vi "Calibration and Function folders.vi"(4 "ini file index":i64, 5 "Folder":T1) -> (2 "error out":errorcluster, 3 "Selected Folder":path)   [LabVIEW 2015]
uses:
  Calibration and Function folders.ctl
  <vilib>/Utility/sysdir.llb/System Directory Type.ctl
panel:
  out "All Files in Dir":path[](array[path])
  out "appended path":path
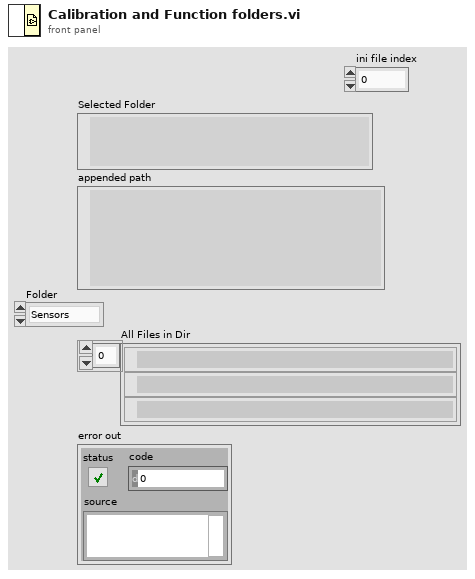
[diagram p1: front panel]
types:
  T1 = typedef "Calibration and Function folders.ctl" = enum16{"Sensors", "Functions", "Config File", "PublicAppFolder", "New ini File", "Set Config File", "Delete ini File"}
  T2 = enum16{"open", "replace", "create", "open or create", "replace or create", "replace or create with confirmation"}
  T3 = typedef "System Directory Type.ctl" = i32
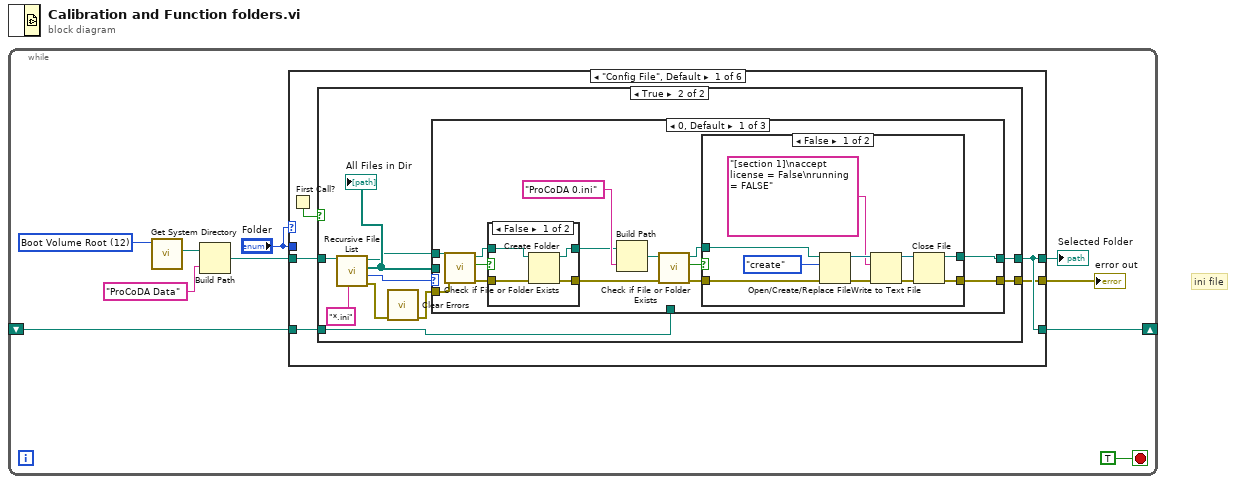
[diagram p0: block diagram]
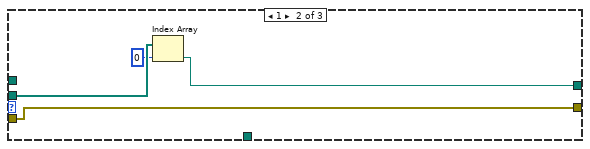
[diagram p5: hidden frame]
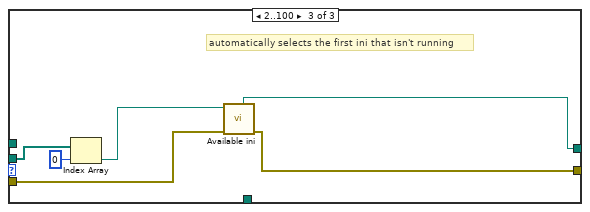
[diagram p6: hidden frame]
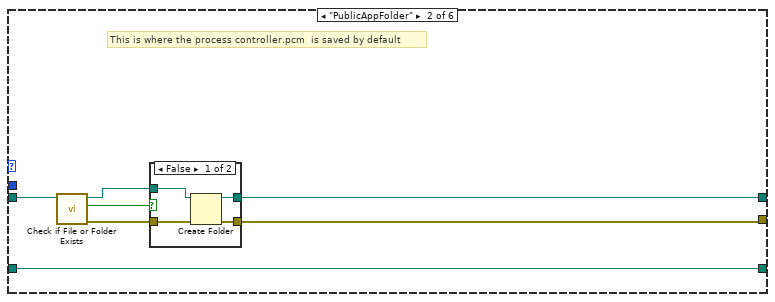
[diagram p7: hidden frame]
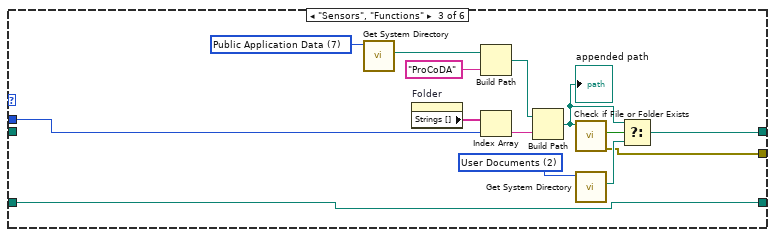
[diagram p9: hidden frame]
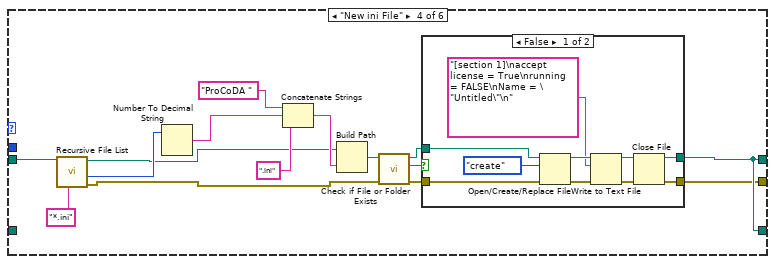
[diagram p10: hidden frame]
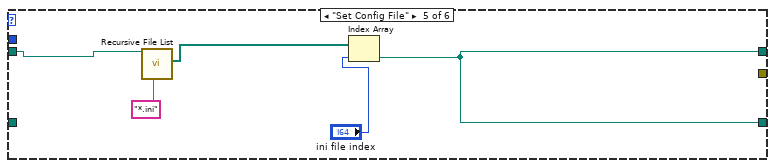
[diagram p12: hidden frame]
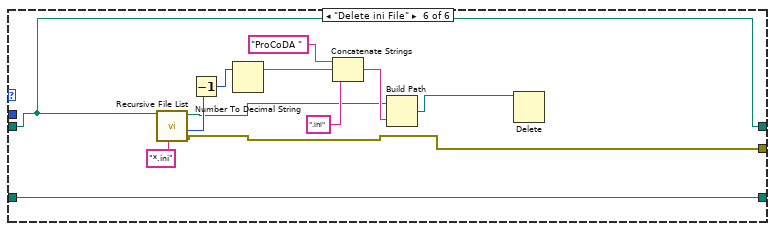
[diagram p13: hidden frame]
diagram:
  # "ini file"
  n1 = while {
    shift-right: [w3] -> _
    shift-left: _ -> [w2]
    stop <- TRUE stop-if-true
    w6 = T3 12 items=["User Home"=0, "User Desktop"=1, "User Documents"=2, "User Application Data"=3, "User Preferences"=4, "User Temporary"=5, "Public Documents"=6, "Public Application Data"=7, "Public Preferences"=8, "Public Cache"=13, "System Core Libraries"=9, "System Installed Libraries"=10, "Application Files"=11, "Boot Volume Root"=12] ("system directory type")
    n2 = call <vilib>:"Get System Directory.vi"("system directory type"=w6) -> ("system directory"=w8:path)  [unwired: 10 in]
    n3 = Build Path(base path=w8, name or relative path="ProCoDA Data") -> (appended path=w5:path)
    n4 = case shown="\"Config File\", Default" "Folder" {
      tunnel: [w14 w72 w90 w108 w123 w128] -> w10
      tunnel: "Folder" -> [_ _ w88 _ _ _]
      tunnel: w5 -> [w15 w71 _ w110 w126 w128]
      tunnel: [w14 w70 w83 w108 w123 w129] -> w3
      tunnel: w2 -> [w12 w70 w83 _ _ w129]
      tunnel: [w13 w69 w82 w107 _ w132] -> w1
      frame "Config File", Default {
        n5 = First Call?() -> (First Call?: T/F=w11:bool)
        n6 = case shown="True" w11 {
          tunnel: w15 -> [_ w26]
          tunnel: [w16 w23] -> w14
          tunnel: [_ w21] -> w13
          tunnel: w12 -> [w16 w18]
          frame False {
          }
          frame True {
            n7 = call <vilib>:"Recursive File List.vi"("pattern"="*.ini", "Folder Path"=w26) -> ("error out"=w19:errorcluster, "Number of Files"=w22:i32, "All Files in Dir"=w24:path[], "dup Folder Path"=w20:path)  [unwired: 5 in, 1 out]
            "All Files in Dir" <- w24
            n8 = call <vilib>:"Clear Errors.vi"("error in (no error)"=w19) -> ("error out"=w17:errorcluster)  [unwired: 5 in, 1 out]
            n9 = case shown="0, Default" w22 {
              tunnel: w24 -> [_ w62 w65]
              tunnel: [w30 w60 w68] -> w23
              tunnel: [w29 w59 w66] -> w21
              tunnel: w20 -> [w28 _ _]
              tunnel: w17 -> [w27 w59 w67]
              tunnel: w18 -> [_ _ _]
              frame 0, Default {
                n10 = call <vilib>:"Check if File or Folder Exists.vi"("error in (no error)"=w27, "path"=w28) -> ("error out"=w38:errorcluster, "file or folder exists?"=w40:bool, "dup path"=w39:path)  [unwired: 7 in]
                n11 = case shown="False" w40 {
                  tunnel: w39 -> [w56 w58]
                  tunnel: w38 -> [w55 w57]
                  tunnel: [w54 w58] -> w36
                  tunnel: [w53 w57] -> w34
                  frame False {
                    n12 = Create Folder(path (use dialog)=w56, error in=w55) -> (created path=w54:path, error out=w53:errorcluster)  [unwired: 1 in, 1 out]
                  }
                  frame True {
                  }
                }
                n13 = Build Path(base path=w36, name or relative path="ProCoDA 0.ini") -> (appended path=w35:path)
                n14 = call <vilib>:"Check if File or Folder Exists.vi"("error in (no error)"=w34, "path"=w35) -> ("error out"=w32:errorcluster, "file or folder exists?"=w33:bool, "dup path"=w31:path)  [unwired: 7 in]
                n15 = case shown="False" w33 {
                  tunnel: w32 -> [w50 w51]
                  tunnel: w31 -> [w49 w52]
                  tunnel: [w47 w52] -> w30
                  tunnel: [w46 w51] -> w29
                  frame False {
                    n16 = Open/Create/Replace File(file path (use dialog)=w49, error in=w50, operation (0:open)=T2."create") -> (refnum out=w43:refnum<file>, error out=w45:errorcluster)  [unwired: 3 in, 1 out]
                    n17 = Write to Text File(file (use dialog)=w43, text="[section 1]\naccept license = False\nrunning = FALSE", error in=w45) -> (refnum out=w42:refnum<file>, error out=w44:errorcluster)  [unwired: 1 in, 1 out]
                    n18 = Close File(refnum=w42, error in=w44) -> (path=w47:path, error out=w46:errorcluster)
                  }
                  frame True {
                  }
                }
              }
              frame 1 {
                n19 = Index Array(array=w62, index=0) -> (element=w60:path)
              }
              frame 2..100 {
                # "automatically selects the first ini that isn't running"
                n20 = Index Array(array=w65, index=0) -> (element=w63:path)
                n21 = call "Available ini.vi"("error in"=w67, "Config file path"=w63) -> ("error out"=w66:errorcluster, "ini file"=w68:path)  [unwired: 4 in, 4 out]
              }
            }
          }
        }
      }
      frame "PublicAppFolder" {
        # "This is where the process controller.pcm  is saved by default"
        n22 = call <vilib>:"Check if File or Folder Exists.vi"("path"=w71) -> ("error out"=w73:errorcluster, "file or folder exists?"=w75:bool, "dup path"=w74:path)  [unwired: 8 in]
        n23 = case shown="False" w75 {
          tunnel: w74 -> [w79 w81]
          tunnel: w73 -> [w78 w80]
          tunnel: [w77 w81] -> w72
          tunnel: [w76 w80] -> w69
          frame False {
            n24 = Create Folder(path (use dialog)=w79, error in=w78) -> (created path=w77:path, error out=w76:errorcluster)  [unwired: 1 in, 1 out]
          }
          frame True {
          }
        }
      }
      frame "Sensors", "Functions" {
        w86 = T3 2 items=["User Home"=0, "User Desktop"=1, "User Documents"=2, "User Application Data"=3, "User Preferences"=4, "User Temporary"=5, "Public Documents"=6, "Public Application Data"=7, "Public Preferences"=8, "Public Cache"=13, "System Core Libraries"=9, "System Installed Libraries"=10, "Application Files"=11, "Boot Volume Root"=12] ("system directory type")
        w95 = T3 7 items=["User Home"=0, "User Desktop"=1, "User Documents"=2, "User Application Data"=3, "User Preferences"=4, "User Temporary"=5, "Public Documents"=6, "Public Application Data"=7, "Public Preferences"=8, "Public Cache"=13, "System Core Libraries"=9, "System Installed Libraries"=10, "Application Files"=11, "Boot Volume Root"=12] ("system directory type")
        n25 = call <vilib>:"Get System Directory.vi"("system directory type"=w95) -> ("system directory"=w85:path)  [unwired: 10 in]
        n26 = property on="Folder" class="Enum (strict)"() -> ("Strings []"=w89:string[])  [unwired: 2 in, 2 out]
        n27 = Build Path(base path=w85, name or relative path="ProCoDA") -> (appended path=w93:path)
        n28 = Index Array(array=w89, index=w88) -> (element=w87:string)
        n29 = Build Path(base path=w93, name or relative path=w87) -> (appended path=w91:path)
        "appended path" <- w91
        n30 = call <vilib>:"Check if File or Folder Exists.vi"("path"=w91) -> ("error out"=w82:errorcluster, "file or folder exists?"=w92:bool)  [unwired: 8 in, 1 out]
        n31 = call <vilib>:"Get System Directory.vi"("system directory type"=w86) -> ("system directory"=w84:path)  [unwired: 10 in]
        n32 = Select(t=w91, s=w92, f=w84) -> (s? t:f=w90:path)
      }
      frame "New ini File" {
        n33 = call <vilib>:"Recursive File List.vi"("pattern"="*.ini", "Folder Path"=w110) -> ("error out"=w96:errorcluster, "Number of Files"=w102:i32, "dup Folder Path"=w97:path)  [unwired: 5 in, 2 out]
        n34 = Number To Decimal String(number=w102) -> (decimal integer string=w100:string)  [unwired: 1 in]
        n35 = Concatenate Strings("ProCoDA " ("name or relative path"), w100, ".ini" ("name or relative path")) -> (w98:string)
        n36 = Build Path(base path=w97, name or relative path=w98) -> (appended path=w106:path)
        n37 = call <vilib>:"Check if File or Folder Exists.vi"("error in (no error)"=w96, "path"=w106) -> ("error out"=w104:errorcluster, "file or folder exists?"=w105:bool, "dup path"=w103:path)  [unwired: 7 in]
        n38 = case shown="False" w105 {
          tunnel: w104 -> [w120 w121]
          tunnel: w103 -> [w119 w122]
          tunnel: [w117 w122] -> w108
          tunnel: [w116 w121] -> w107
          frame False {
            n39 = Open/Create/Replace File(file path (use dialog)=w119, error in=w120, operation (0:open)=T2."create") -> (refnum out=w113:refnum<file>, error out=w115:errorcluster)  [unwired: 3 in, 1 out]
            n40 = Write to Text File(file (use dialog)=w113, text="[section 1]\naccept license = True\nrunning = FALSE\nName = \"Untitled\"\n", error in=w115) -> (refnum out=w112:refnum<file>, error out=w114:errorcluster)  [unwired: 1 in, 1 out]
            n41 = Close File(refnum=w112, error in=w114) -> (path=w117:path, error out=w116:errorcluster)
          }
          frame True {
          }
        }
      }
      frame "Set Config File" {
        n42 = call <vilib>:"Recursive File List.vi"("pattern"="*.ini", "Folder Path"=w126) -> ("All Files in Dir"=w125:path[])  [unwired: 5 in, 4 out]
        n43 = Index Array(array=w125, index="ini file index") -> (element=w123:path)
      }
      frame "Delete ini File" {
        n44 = call <vilib>:"Recursive File List.vi"("pattern"="*.ini", "Folder Path"=w128) -> ("error out"=w132:errorcluster, "Number of Files"=w138:i32, "dup Folder Path"=w133:path)  [unwired: 5 in, 2 out]
        n45 = Decrement(x=w138) -> (x-1=w131:i32)
        n46 = Number To Decimal String(number=w131) -> (decimal integer string=w136:string)  [unwired: 1 in]
        n47 = Concatenate Strings("ProCoDA " ("name or relative path"), w136, ".ini" ("name or relative path")) -> (w134:string)
        n48 = Build Path(base path=w133, name or relative path=w134) -> (appended path=w130:path)
        n49 = Delete(path (use dialog)=w130) -> ()  [unwired: 4 in, 3 out]
      }
    }
    "Selected Folder" <- w10
    "error out" <- w1
  }
